vi "parse string to end of line.vi"(8 "error in (no error)":errorcluster, 11 "String":string) -> (0 "error out":errorcluster, 3 "string to eol":string)   [LabVIEW 2013]
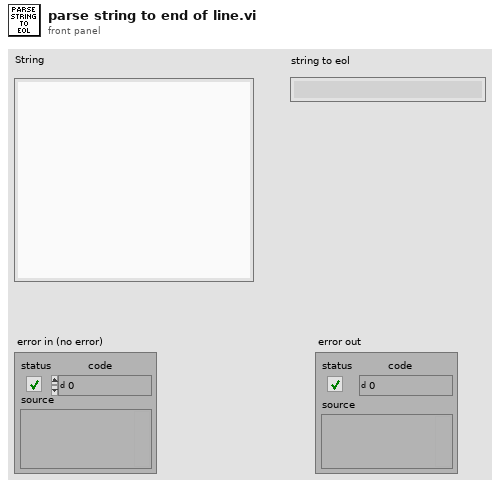
[diagram p1: front panel]
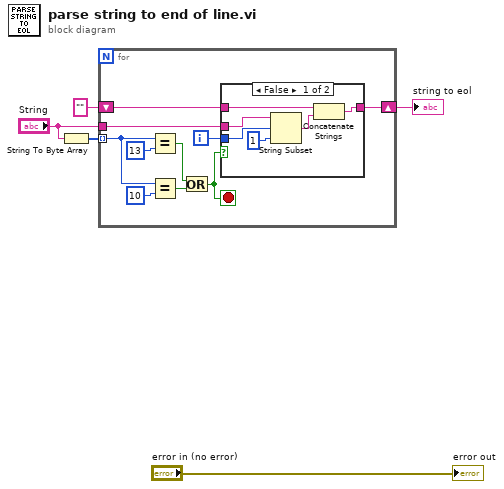
[diagram p0: block diagram]
diagram:
  n1 = String To Byte Array(string="String") -> (unsigned byte array=w5:u8[])
  n2 = for {
    tunnel: w5 -> [w14] mode=indexing
    shift-right: [w7] -> w2
    shift-left: "" -> [w8]
    tunnel: "String" -> [w10]
    i -> [w9]
    stop <- w6 stop-if-true
    n3 = Equal?(x=w14, y=u8 13) -> (x = y?=w12:bool)
    n4 = Equal?(x=w14, y=u8 10) -> (x = y?=w11:bool)
    n5 = Or(x=w12, y=w11) -> (x .or. y?=w6:bool)
    n6 = case shown="False" w6 {
      tunnel: w10 -> [w21 _]
      tunnel: w9 -> [w20 _]
      tunnel: w8 -> [w18 w22]
      tunnel: [w16 w22] -> w7
      frame False {
        n7 = String Subset(string=w21, offset (0)=w20, length (rest)=1 ("length (rest)")) -> (substring=w17:string)
        n8 = Concatenate Strings(w18, w17) -> (w16:string)
      }
      frame True {
      }
    }
  }
  "string to eol" <- w2
  "error out" <- "error in (no error)"
